vi "SDCP - Standard Message Frames Editor - Update Parameter List Table.vi"(3 "error in (no error)":errorcluster, 4 "Listbox reference":refnum<vi>, 5 "Input frame list":T2(array[cluster])) -> (0 "error out":errorcluster)   [LabVIEW 2020]
uses:
  Typedefs/SDCP - Standard Message Frames Editor - Parameter cluster.ctl
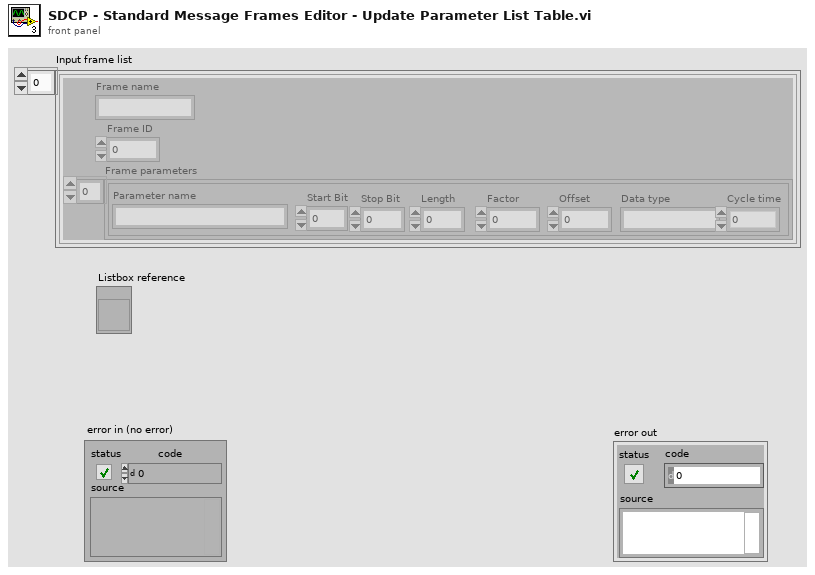
[diagram p1: front panel]
types:
  T1 = typedef "SDCP - Standard Message Frames Editor - Parameter cluster.ctl" = cluster{"Parameter name":string, "Start Bit":i32, "Stop Bit":i32, "Length":i32, "Factor":dbl, "Offset":dbl, "Data type":string, "Cycle time":dbl}
  T2 = cluster{"Frame name":string, "Frame ID":i32, "Frame parameters":T1[]}[]
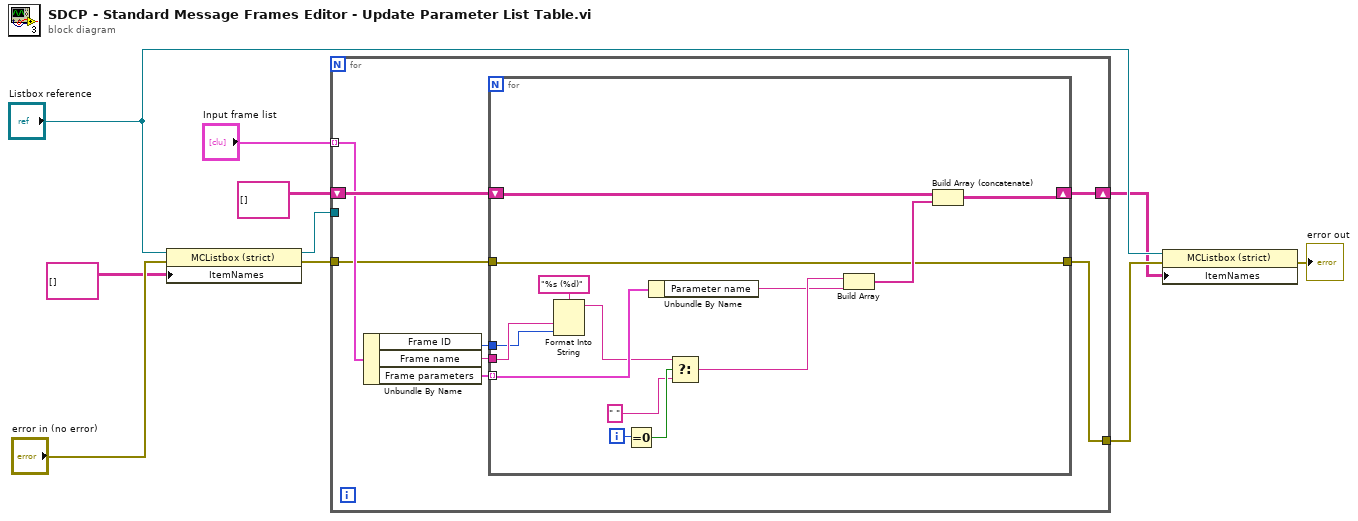
[diagram p0: block diagram]
diagram:
  n1 = property class="MCListbox (strict)"(reference="Listbox reference", error in="error in (no error)", "ItemNames"=string[][] [] ("Item Names")) -> (reference out=w5:refnum<vi>, error out=w6:errorcluster)
  n2 = for {
    tunnel: "Input frame list" -> [w17] mode=indexing
    shift-right: [w14] -> w2
    shift-left: string[][] [] -> [w18]
    tunnel: w6 -> [w13]
    tunnel: w5 -> [_]
    tunnel: [w12] -> w4
    n3 = Unbundle By Name(w17) -> ("Frame ID"=w11:i32, "Frame name"=w15:string, "Frame parameters"=w16:T1[])
    n4 = for {
      shift-right: [w24] -> w14
      shift-left: w18 -> [w26]
      tunnel: w16 -> [w28] mode=indexing
      tunnel: w15 -> [w21]
      tunnel: w13 -> [w23]
      tunnel: [w23] -> w12
      tunnel: w11 -> [w20]
      i -> [w32]
      n5 = Format Into String(format string="%s (%d)", w21, w20) -> (resulting string=w19:string)  [unwired: 2 in, 1 out]
      n6 = Equal To 0?(x=w32) -> (x = 0?=w31:bool)
      n7 = Unbundle By Name(w28) -> ("Parameter name"=w27:string)
      n8 = Select(t=w19, s=w31, f=" ") -> (s? t:f=w29:string)
      n9 = Build Array(w29, w27) -> (w25:string[])
      n10 = Build Array (concatenate)(w26, w25) -> (w24:string[][])
    }
  }
  n11 = property class="MCListbox (strict)"(reference="Listbox reference", error in=w4, "ItemNames"=w2) -> (error out=→"error out":errorcluster)  [unwired: 1 out]
